vi "MD Select 1D DBL.vi"(5 "First Array":dbl[](array[numeric]), 7 "Condition":bool[](array[boolean]), 9 "Second Array":dbl[](array[numeric])) -> (8 "Resulting Array":dbl[](array[numeric]))   [LabVIEW 2011, in "Super Simple Neural Network.lvlib"]
doc: "Select the first array element if the codition is True. If the condition is False select the second array element. The arrays should be the same size."
uses:
  Super Simple Neural Network.lvlib
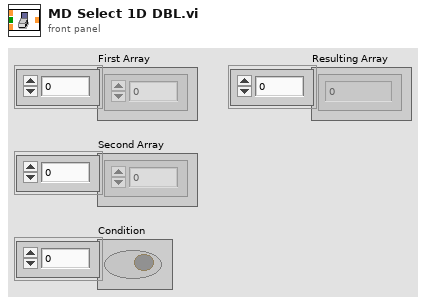
[diagram p1: front panel]
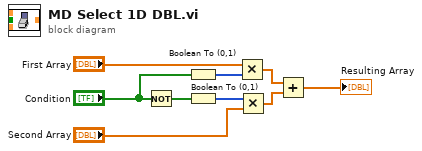
[diagram p0: block diagram]
diagram:
  n1 = Not(x="Condition") -> (.not. x?=w2:bool[])
  n2 = Boolean To (0,1)(Boolean="Condition") -> (0, 1=w3:i16[])
  n3 = Boolean To (0,1)(Boolean=w2) -> (0, 1=w5:i16[])
  n4 = Multiply(x="First Array", y=w3) -> (x*y=w7:dbl[])
  n5 = Multiply(x=w5, y="Second Array") -> (x*y=w8:dbl[])
  n6 = Add(x=w7, y=w8) -> (x+y=→"Resulting Array":dbl[])
